vi "DropVI_SimpleClientSubscriber.vi"() -> ()   [LabVIEW 2013, in "MQTT Client.lvlib"]
uses:
  MQTT Client.lvlib
  <vilib>/LabVIEW Open Source Project/MQTT Connection/MQTT_Connection/Connection/Connection.lvclass
  Client class/Client.lvclass/Client.ctl
  <vilib>/LabVIEW Open Source Project/MQTT Connection/MQTT_Base/Base Class/MQTT_Base.lvclass/MQTT_Base.ctl
  <vilib>/LabVIEW Open Source Project/MQTT Control Packets/Control Packets/PUBLISH/PUBLISH.lvclass
  Client class/Client.lvclass
  <vilib>/LabVIEW Open Source Project/MQTT Connection/MQTT_Base/Base Class/MQTT_Base.lvclass
panel:
  out "last error":errorcluster
  out "Unsuback":bool
  in  "Subscribe":bool
  in  "Connection":bool
  out "Waveform Chart":dbl(graph)
  out "Suback":bool
  in  "Stop Client":bool
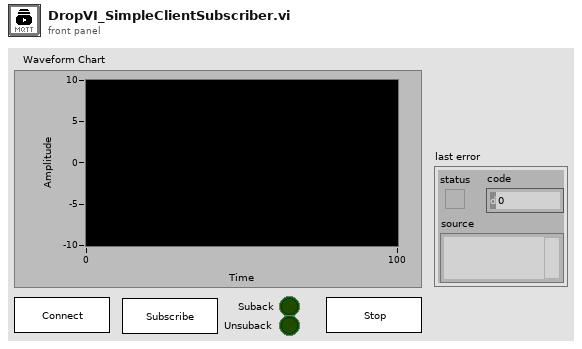
[diagram p1: front panel]
types:
  T1 = typedef "MQTT Client.lvlib/Client.lvclass/Public Events -- cluster.ctl" = cluster{"Connection Status":refnum<user-event>, "Connected":refnum<user-event>, "Application Message":refnum<user-event>}
  T2 = typedef "MQTT Base.lvlib/MQTT_Base.lvclass/Public Events -- cluster.ctl" = cluster{"Stop Event":refnum<user-event>, "Error Event":refnum<user-event>, "Inbound Message":refnum<user-event>}
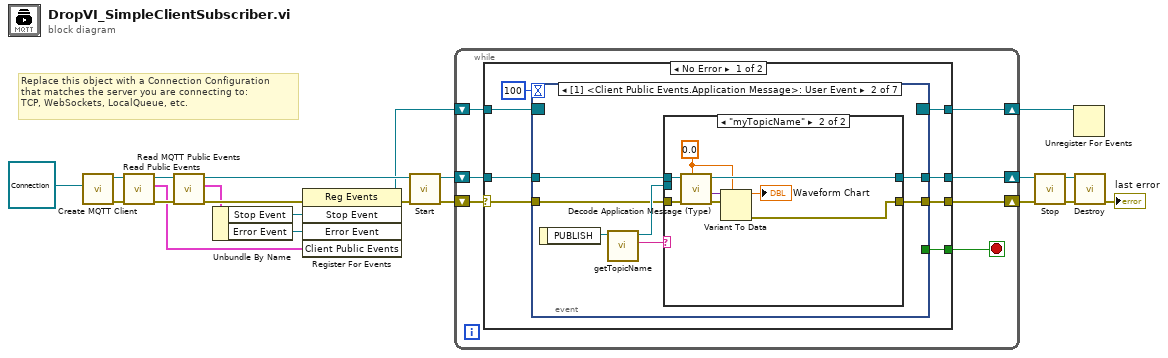
[diagram p0: block diagram]
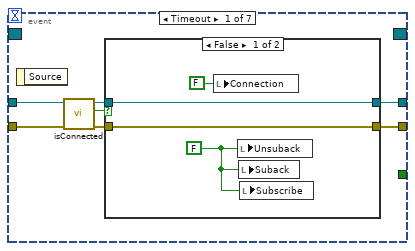
[diagram p2: hidden frame]
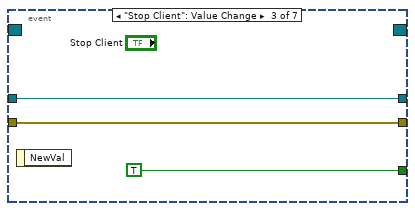
[diagram p5: hidden frame]
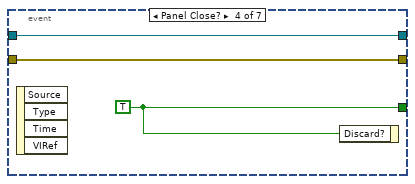
[diagram p6: hidden frame]
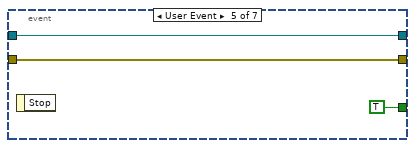
[diagram p7: hidden frame]
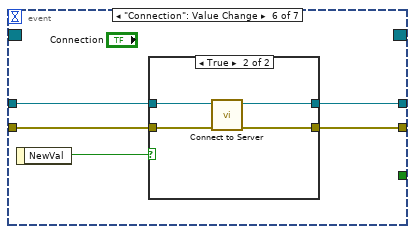
[diagram p8: hidden frame]
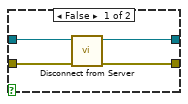
[diagram p9: hidden frame]
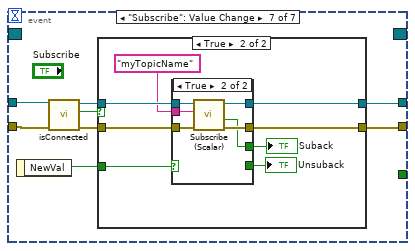
[diagram p10: hidden frame]
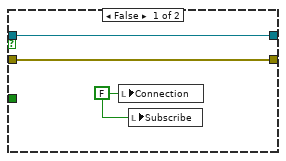
[diagram p11: hidden frame]
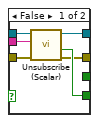
[diagram p12: hidden frame]
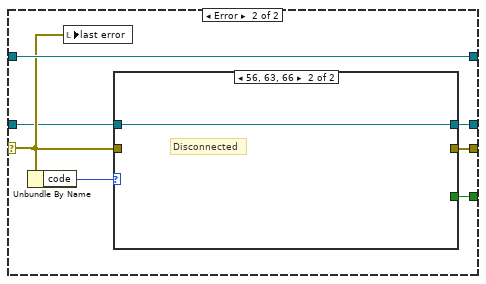
[diagram p13: hidden frame]
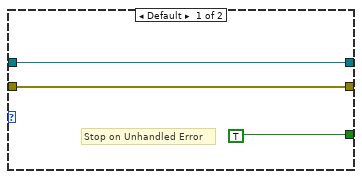
[diagram p14: hidden frame]
diagram:
  # "Replace this object with a Connection Configuration\nthat matches the server you are connecting to:\nTCP, WebSockets, LocalQueue, etc."
  n1 = call "Create MQTT Client.vi"("Connection Configuration"=refnum<class "Connection.lvclass"> refnum) -> ("error out"=w19:errorcluster, "Client out"=w21:refnum<class "Client.lvclass">)  [unwired: 9 in]
  n2 = call "Read Public Events.vi"("error in (no error)"=w19, "Client in"=w21) -> ("error out"=w18:errorcluster, "Client Public Events"=w16:T1, "Client out"=w20:refnum<class "Client.lvclass">)  [unwired: 7 in]
  n3 = call <vilib>:"Read MQTT Public Events.vi"("error in (no error)"=w18, "MQTT_Base in"=w20) -> ("error out"=w17:errorcluster, "MQTT Public Events"=w9:T2, "MQTT_Base out"=w14:refnum<class "Client.lvclass">)  [unwired: 7 in]
  n4 = Unbundle By Name(w9) -> ("Stop Event"=w11:refnum<user-event>, "Error Event"=w10:refnum<user-event>)
  n5 = register-events(error in=w17, w11, w10, w16) -> (reference out=w13:refnum<event-registration>, error out=w15:errorcluster)  [unwired: 1 in]
  n6 = call <vilib>:"Start.vi"("error in (no error)"=w15, "MQTT_Base in"=w14) -> ("error out"=w2:errorcluster, "MQTT_Base out"=w3:refnum<class "Client.lvclass">)  [unwired: 7 in, 1 out]
  n7 = while {
    shift-right: [w27] -> w12
    shift-left: w13 -> [w28]
    shift-right: [w24] -> w6
    shift-left: w3 -> [w25]
    shift-right: [w26] -> w4
    shift-left: w2 -> [w22]
    stop <- w23 stop-if-true
    n8 = case shown="No Error" w22 {
      selector: w22 -> [w29 w123]
      tunnel: w28 -> [w36 w126]
      tunnel: [w35 w126] -> w27
      tunnel: [w34 w121] -> w26
      tunnel: w25 -> [w32 w122]
      tunnel: [w31 w125] -> w24
      tunnel: [w30 w120] -> w23
      frame No Error {
        n9 = event shown="[1] <Client Public Events.Application Message>: User Event" {
          selector: w36 -> [_ _ _ _ _ _ _]
          dyn-events: [_ _ _ _ _ _ _] -> w35
          timeout: 100 -> [_ _ _ _ _ _ _]
          tunnel: w29 -> [w39 w53 w68 w70 w75 w76 w94]
          tunnel: [w42 w50 w68 w70 w75 w77 w95] -> w34
          tunnel: [_ _ TRUE w72 TRUE _ _] -> w30
          tunnel: w32 -> [w41 w54 w69 w71 w73 w80 w93]
          tunnel: [w43 w52 w69 w71 w73 w78 w96] -> w31
          event Timeout {
            n10 = event-data() -> ()  [unwired: 1 in, 1 out]
            n11 = call "isConnected.vi"("error in (no error)"=w39, "Client in"=w41) -> ("error out"=w38:errorcluster, "connected"=w37:bool, "Client out"=w40:refnum<class "Client.lvclass">)  [unwired: 7 in]
            n12 = case shown="False" w37 {
              tunnel: [w47 w49] -> w43
              tunnel: [w46 w48] -> w42
              tunnel: w40 -> [w47 w49]
              tunnel: w38 -> [w46 w48]
              frame False {
                w45 = FALSE
                n13 = local write "Connection"(FALSE ("Connection")) -> ()
                n14 = local write "Unsuback"(w45) -> ()
                n15 = local write "Suback"(w45) -> ()
                n16 = local write "Subscribe"(w45) -> ()
              }
              frame True {
              }
            }
          }
          event User Event {
            n17 = event-data() -> ("PUBLISH"=w56:refnum<class "PUBLISH.lvclass">)  [unwired: 1 in]
            n18 = call <vilib>:"getTopicName.vi"("PUBLISH in"=w56) -> ("Topic"=w51:string, "PUBLISH out"=w55:refnum<class "PUBLISH.lvclass">)  [unwired: 8 in, 1 out]
            n19 = case shown="\"myTopicName\"" w51 {
              tunnel: w55 -> [_ _]
              tunnel: w54 -> [w58 w64]
              tunnel: w53 -> [w57 w62]
              tunnel: [w58 w63] -> w52
              tunnel: [w57 w66] -> w50
              frame Default {
              }
              frame "myTopicName" {
                w60 = 0.0
                n20 = call "Decode Application Message (Type).vi"("Type"=w60, "error in (no error)"=w62, "Client in"=w64) -> ("error out"=w61:errorcluster, "Payload"=w59:variant, "Client out"=w63:refnum<class "Client.lvclass">)  [unwired: 5 in, 1 out]
                n21 = Variant To Data(error in=w61, type=w60, Variant=w59) -> (data=→"Waveform Chart":dbl, error out=w66:errorcluster)
              }
            }
          }
          event "Stop Client": Value Change {
            n22 = event-data() -> ()  [unwired: 1 in, 1 out]
          }
          event Panel Close? {
            w72 = TRUE
            n23 = event-data() -> ()  [unwired: 1 in, 4 out]
            n24 = event-data("Discard?"=w72) -> ()  [unwired: 1 in, 1 out]
          }
          event User Event {
            n25 = event-data() -> ()  [unwired: 1 in, 1 out]
          }
          event "Connection": Value Change {
            n26 = event-data() -> ("NewVal"=w79:bool)  [unwired: 1 in]
            n27 = case shown="True" w79 {
              tunnel: w80 -> [w84 w88]
              tunnel: [w83 w85] -> w78
              tunnel: [w82 w86] -> w77
              tunnel: w76 -> [w81 w87]
              frame False {
                n28 = call "Disconnect from Server.vi"("error in (no error)"=w81, "Client in"=w84) -> ("error out"=w82:errorcluster, "Client out"=w83:refnum<class "Client.lvclass">)  [unwired: 7 in, 1 out]
              }
              frame True {
                n29 = call "Connect to Server.vi"("error in (no error)"=w87, "Client in"=w88) -> ("error out"=w86:errorcluster, "Client out"=w85:refnum<class "Client.lvclass">)  [unwired: 6 in, 2 out]
              }
            }
          }
          event "Subscribe": Value Change {
            n30 = event-data() -> ("NewVal"=w89:bool)  [unwired: 1 in]
            n31 = call "isConnected.vi"("error in (no error)"=w94, "Client in"=w93) -> ("error out"=w91:errorcluster, "connected"=w90:bool, "Client out"=w92:refnum<class "Client.lvclass">)  [unwired: 7 in]
            n32 = case shown="True" w90 {
              tunnel: [w99 w107] -> w96
              tunnel: [w98 w106] -> w95
              tunnel: w92 -> [w99 w105]
              tunnel: w91 -> [w98 w104]
              tunnel: w89 -> [_ w102]
              frame False {
                w97 = FALSE ("Connection")
                n33 = local write "Connection"(w97) -> ()
                n34 = local write "Subscribe"(w97) -> ()
              }
              frame True {
                n35 = case shown="True" w102 {
                  tunnel: [w108 w116] -> w107
                  tunnel: [w109 w115] -> w106
                  tunnel: w105 -> [w113 w119]
                  tunnel: w104 -> [w112 w118]
                  tunnel: "myTopicName" ("Topic Name (empty: Payload name)") -> [w111 w117]
                  tunnel: [_ w114] -> w101
                  tunnel: [w110 _] -> w100
                  frame False {
                    n36 = call "Unsubscribe (Scalar).vi"("error in (no error)"=w112, "Topic Filter"=w111, "Client in"=w113) -> ("error out"=w109:errorcluster, "Ack"=w110:bool, "Client out"=w108:refnum<class "Client.lvclass">)  [unwired: 6 in]
                  }
                  frame True {
                    n37 = call "Subscribe (Scalar).vi"("error in (no error)"=w118, "Topic Filter"=w117, "Client in"=w119) -> ("error out"=w115:errorcluster, "Ack"=w114:bool, "Client out"=w116:refnum<class "Client.lvclass">)  [unwired: 6 in]
                  }
                }
                "Unsuback" <- w100
                "Suback" <- w101
              }
            }
          }
        }
      }
      frame Error {
        n38 = Unbundle By Name(w123) -> ("code"=w124:i32)
        n39 = local write "last error"(w123) -> ()
        n40 = case shown="56, 63, 66" w124 {
          tunnel: w122 -> [w129 w130]
          tunnel: [w129 w130] -> w125
          tunnel: w123 -> [w128 _]
          tunnel: [w128 _] -> w121
          tunnel: [TRUE _] -> w120
          frame Default {
            # "Stop on Unhandled Error"
          }
          frame 56, 63, 66 {
            # "Disconnected"
          }
        }
      }
    }
  }
  n41 = call <vilib>:"Stop.vi"("error in (no error)"=w4, "MQTT_Base in"=w6) -> ("error out"=w5:errorcluster, "MQTT_Base out"=w7:refnum<class "Client.lvclass">)  [unwired: 7 in, 1 out]
  n42 = Unregister For Events(event registration refnum=w12) -> ()  [unwired: 1 in, 1 out]
  n43 = call <vilib>:"Destroy.vi"("error in (no error)"=w5, "MQTT_Base in"=w7) -> ("error out"=→"last error":errorcluster)  [unwired: 8 in, 1 out]
